vi "SetSinglePoint.vi"() -> ()   [LabVIEW 2010]
uses:
  NI Modbus.llb/MB Serial Master Query Write Single Register (poly).vi
  ModBUS Driver/Private/MBDRV_Action.ctl
  ModBUS Driver/Private/MBDRV_Command Data.ctl
  ModBUS Driver/Private/MBDRV_Command List.ctl
  Drivers/ModbusServer/DeviceListChannelData.ctl
  Drivers/ModbusServer/AutoChannelData.ctl
panel:
  in  "SP2":dbl caption="设置点2" format="%.1f"
  in  "SP1":dbl caption="设置点1" format="%.1f"
  in  "OK":bool
  in  "Cancel":bool
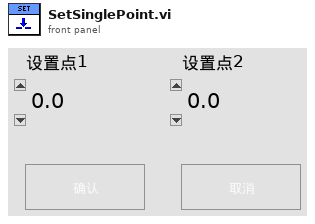
[diagram p1: front panel]
types:
  T1 = cluster{"Mode":enum16{"RTU", "ASCII"}, "Slave Address":u8}
  T2 = typedef "MBDRV_Command Data.ctl" = cluster{"Action":T3, "Com Port":string, "Register Address":u16, "Data To Write/Num To Read":i16}
  T3 = typedef "MBDRV_Action.ctl" = enum16{"Write", "Read"}
  T4 = typedef "Path InitPaths__FS.ctl" = cluster{"Ctrller CFG":path, "INI":path, "Profile":path, "EventLog":path, "Data":path}
  T5 = typedef "Controller Configuration__CHC.ctl" = cluster{"Ctrller Type":T6, "Ctrller Name":string, "Ctrller Addr":string, "Server IP":string, "Conn Result":string, "Port":string, "Baud":dbl}
  T6 = typedef "Controller Configuration__Ctrller Type.ctl" = enum16{"F4S/D", "Synergy"}
  T7 = typedef "MBDRV_Command List.ctl" = T2[]
  T8 = typedef "MonitorServer.lvlib/DeviceListChannelData.ctl" = T9[]
  T9 = typedef "MonitorServer.lvlib/AutoChannelData.ctl" = cluster{"DeviceName":string, "Channel1":dbl, "SetPoint1":dbl, "Channel2":dbl, "SetPoint2":dbl, "ConnectOK":bool, "DecimalPoint1":i16, "DecimalPoint2":i16}
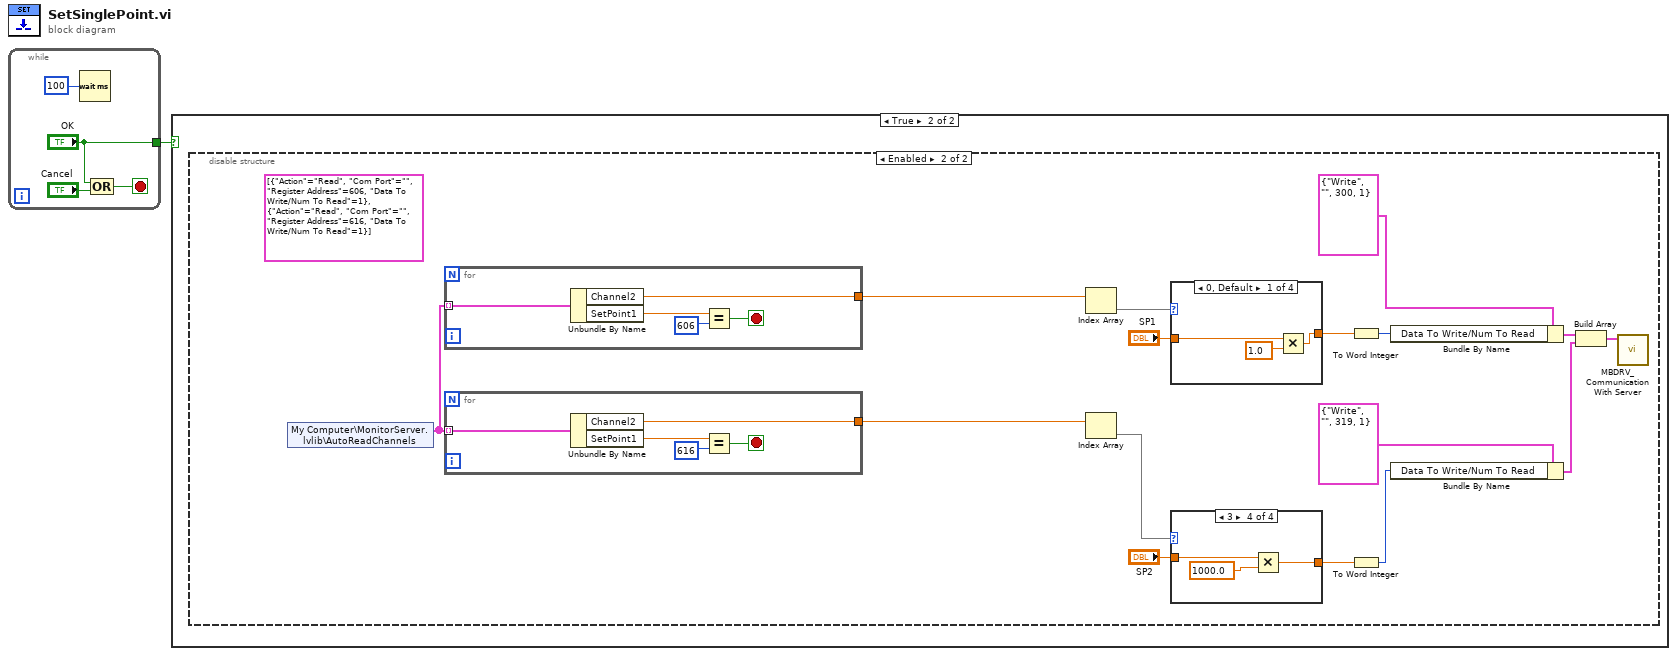
[diagram p0: block diagram]
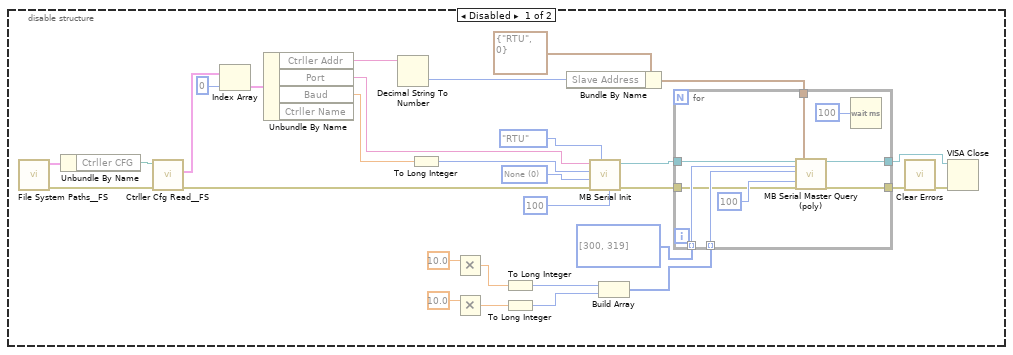
[diagram p3: hidden frame]
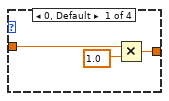
[diagram p4: hidden frame]
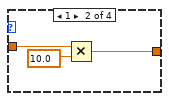
[diagram p5: hidden frame]
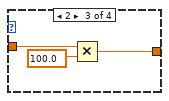
[diagram p6: hidden frame]
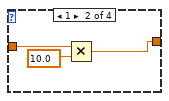
[diagram p7: hidden frame]
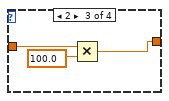
[diagram p8: hidden frame]
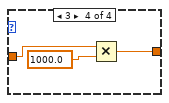
[diagram p9: hidden frame]
diagram:
  n1 = while {
    tunnel: ["OK"] -> w1
    stop <- w4 stop-if-true
    n2 = Wait (ms)(milliseconds to wait=u32 100) -> ()  [unwired: 1 out]
    n3 = Compound Arithmetic op=OR("OK", "Cancel") -> (w4:bool)
  }
  n4 = case shown="True" w1 {
    frame False {
    }
    frame True {
      n5 = disable-structure shown="Enabled" {
        frame Disabled {
          w11 = u16 0 items=["None", "Odd", "Even", "Mark", "Space"] ("Parity")
          n6 = call "File System Paths__FS.vi"() -> ("error out"=w14:errorcluster, "FilePaths"=w20:T4)  [unwired: 9 in, 1 out]
          n7 = Unbundle By Name(w20) -> ("Ctrller CFG"=w21:path)
          n8 = call "Ctrller Cfg Read__FS.vi"("error in (no error)"=w14, "Path In"=w21) -> ("error out"=w7:errorcluster, "Ctrllers"=w19:T5[])  [unwired: 7 in, 1 out]
          n9 = Index Array(array=w19, index=0) -> (element=w17:T5)
          n10 = Unbundle By Name(w17) -> ("Ctrller Addr"=w16:string, "Port"=w10:string, "Baud"=w15:dbl)  [unwired: 1 out]
          n11 = Decimal String To Number(string=w16) -> (number=w8:i32)  [unwired: 2 in, 1 out]
          n12 = To Long Integer(number=w15) -> (32bit integer=w12:i32)
          n13 = Multiply(x=10.0) -> (x*y=w27:dbl)  [unwired: 1 in]
          n14 = Multiply(x=10.0) -> (x*y=w23:dbl)  [unwired: 1 in]
          n15 = To Long Integer(number=w27) -> (32bit integer=w25:i32)
          n16 = To Long Integer(number=w23) -> (32bit integer=w22:i32)
          n17 = Bundle By Name(cluster=T1 {"Mode"=enum."RTU", "Slave Address"=0} ("Serial Parameters"), "Slave Address"=w8) -> (w31:T1)
          n18 = call "MB Serial Init.vi"("Timeout"=u32 100, "Mode"=enum16{"RTU", "ASCII"}."RTU", "error in (no error)"=w7, "Parity"=w11, "Baud Rate"=w12, "VISA resource name"=w10) -> ("error out"=w32:errorcluster, "VISA resource name out"=w33:refnum<visa-resource-name>)  [unwired: 4 in]
          n19 = Build Array(w25, w22) -> (w34:i32[])
          n20 = for {
            tunnel: u16[] [300, 319] ("Regs Address") -> [w44] mode=indexing
            tunnel: w34 -> [w43] mode=indexing
            tunnel: w33 -> [w42]
            tunnel: w32 -> [w39]
            tunnel: [w38] -> w30
            tunnel: [w37] -> w29
            tunnel: w31 -> [w36]
            n21 = call-poly "MB Serial Master Query (poly).vi"("VISA resource name"=w42, "Address"=w44, "Holding Register"=w43, "Timeout"=u32 100, "error in"=w39, "Serial Parameters"=w36) -> ("VISA resource name out"=w37:refnum<visa-resource-name>, "error out"=w38:errorcluster)  [unwired: 11 in, 1 out]
            n22 = Wait (ms)(milliseconds to wait=u32 100) -> ()  [unwired: 1 out]
          }
          n23 = call <vilib>:"Clear Errors.vi"("error in (no error)"=w30) -> ("error out"=w28:errorcluster)  [unwired: 6 in]
          n24 = VISA Close(VISA resource name=w29, error in (no error)=w28) -> ()  [unwired: 1 out]
        }
        frame Enabled {
          (unwired) T7 [{"Action"=enum."Read", "Com Port"="", "Register Address"=606, "Data To Write/Num To Read"=1}, {"Action"=enum."Read", "Com Port"="", "Register Address"=616, "Data To Write/Num To Read"=1}] ("Command List")
          n25 = shared-variable "My Computer\\MonitorServer.lvlib\\AutoReadChannels"() -> (w57:T8)  [unwired: 1 in, 1 out]
          n26 = for {
            tunnel: w57 -> [w82] mode=indexing
            tunnel: [w78] -> w60
            stop <- w79 stop-if-true
            n27 = Unbundle By Name(w82) -> ("Channel2"=w78:dbl, "SetPoint1"=w81:dbl)
            n28 = Equal?(x=w81, y=u16 606 ("Register Address")) -> (x = y?=w79:bool)
          }
          n29 = for {
            tunnel: w57 -> [w77] mode=indexing
            tunnel: [w73] -> w56
            stop <- w74 stop-if-true
            n30 = Unbundle By Name(w77) -> ("Channel2"=w73:dbl, "SetPoint1"=w76:dbl)
            n31 = Equal?(x=w76, y=616 ("Register Address")) -> (x = y?=w74:bool)
          }
          n32 = Index Array(array=w60) -> (element=w59)  [unwired: 1 in]
          n33 = Index Array(array=w56) -> (element=w55)  [unwired: 1 in]
          n34 = case shown="0, Default" w59 {
            tunnel: [w84 w87 w90 w93] -> w52
            tunnel: "SP1" -> [w83 w86 w89 w92]
            frame 0, Default {
              n35 = Multiply(x=w83, y=1.0) -> (x*y=w84:dbl)
            }
            frame 1 {
              n36 = Multiply(x=w86, y=10.0) -> (x*y=w87:dbl)
            }
            frame 2 {
              n37 = Multiply(x=w89, y=100.0) -> (x*y=w90:dbl)
            }
            frame 3 {
              n38 = Multiply(x=w92, y=1000.0) -> (x*y=w93:dbl)
            }
          }
          n39 = case shown="3" w55 {
            tunnel: [w62 w65 w68 w71] -> w53
            tunnel: "SP2" -> [w61 w64 w67 w70]
            frame 0, Default {
              n40 = Multiply(x=w61, y=1.0) -> (x*y=w62:dbl)
            }
            frame 1 {
              n41 = Multiply(x=w64, y=10.0) -> (x*y=w65:dbl)
            }
            frame 2 {
              n42 = Multiply(x=w67, y=100.0) -> (x*y=w68:dbl)
            }
            frame 3 {
              n43 = Multiply(x=w70, y=1000.0) -> (x*y=w71:dbl)
            }
          }
          n44 = To Word Integer(number=w52) -> (16bit integer=w50:i16)
          n45 = To Word Integer(number=w53) -> (16bit integer=w48:i16)
          n46 = Bundle By Name(cluster=T2 {"Action"=enum."Write", "Com Port"="", "Register Address"=300, "Data To Write/Num To Read"=1} ("Command"), "Data To Write/Num To Read"=w50) -> (w47:T2)
          n47 = Bundle By Name(cluster=T2 {"Action"=enum."Write", "Com Port"="", "Register Address"=319, "Data To Write/Num To Read"=1} ("Command"), "Data To Write/Num To Read"=w48) -> (w46:T2)
          n48 = Build Array(w47, w46) -> (w45:T2[])
          n49 = call "MBDRV_Communication With Server.vi"("Write To PLC"=w45) -> ()  [unwired: 9 in, 2 out]
        }
      }
    }
  }
